vi "Pressure converstion.vi"(0 "Mod2/AI9":fxp<+/-,24,5>, 1 "Mod2/AI8":fxp<+/-,24,5>, 2 "Mod2/AI7":fxp<+/-,24,5>, 5 "Mod2/AI15":fxp<+/-,24,5>, 7 "Mod2/AI10":fxp<+/-,24,5>, 9 "Mod2/AI14":fxp<+/-,24,5>, 12 "Mod2/AI11":fxp<+/-,24,5>, 13 "Mod2/AI12":fxp<+/-,24,5>, 14 "Mod2/AI13":fxp<+/-,24,5>) -> (4 "P8 toP16":fxp<+/-,48,10>[](array[numeric]))   [LabVIEW 2018]
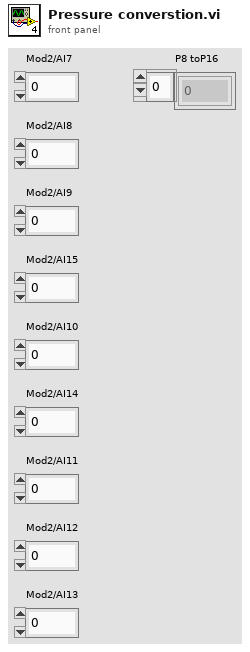
[diagram p1: front panel]
types:
  T1 = cluster{"Gain":fxp<+/-,24,5>, "offset":fxp<+/-,24,5>}
  T2 = cluster{"Gain":fxp<+/-,24,5>, "offset":fxp<+/-,24,5>, "offset 2":fxp<+/-,24,5>}
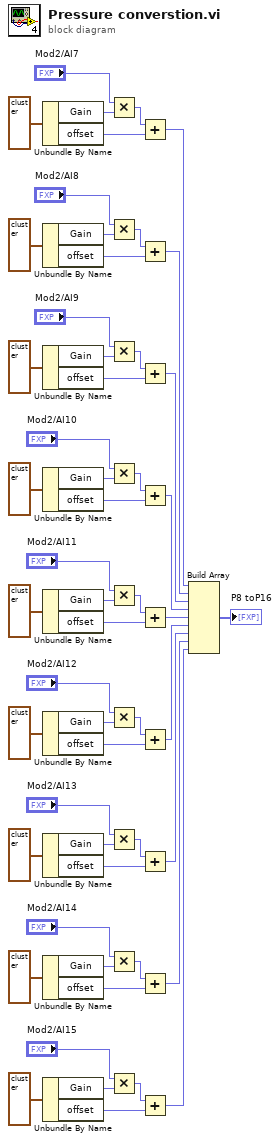
[diagram p0: block diagram]
diagram:
  n1 = Unbundle By Name(T1 {"Gain"=1.0, "offset"=0.0} ("Share_8_P")) -> ("Gain"=w25:fxp<+/-,24,5>, "offset"=w26:fxp<+/-,24,5>)
  n2 = Unbundle By Name(T1 {"Gain"=1.0, "offset"=0.0} ("Share_9_P")) -> ("Gain"=w27:fxp<+/-,24,5>, "offset"=w28:fxp<+/-,24,5>)
  n3 = Unbundle By Name(T1 {"Gain"=1.0, "offset"=0.0} ("Share_10_P")) -> ("Gain"=w29:fxp<+/-,24,5>, "offset"=w30:fxp<+/-,24,5>)
  n4 = Unbundle By Name(T1 {"Gain"=1.0, "offset"=0.0} ("Share_11_P")) -> ("Gain"=w31:fxp<+/-,24,5>, "offset"=w32:fxp<+/-,24,5>)
  n5 = Unbundle By Name(T1 {"Gain"=1.0, "offset"=0.0} ("Share_12_P")) -> ("Gain"=w33:fxp<+/-,24,5>, "offset"=w34:fxp<+/-,24,5>)
  n6 = Unbundle By Name(T1 {"Gain"=1.0, "offset"=0.0} ("Share_13_P")) -> ("Gain"=w35:fxp<+/-,24,5>, "offset"=w36:fxp<+/-,24,5>)
  n7 = Unbundle By Name(T2 {"Gain"=1.0, "offset"=0.0, "offset 2"=0.0} ("Share_14_P")) -> ("Gain"=w37:fxp<+/-,24,5>, "offset"=w38:fxp<+/-,24,5>)
  n8 = Unbundle By Name(T1 {"Gain"=1.0, "offset"=0.0} ("Share_15_P")) -> ("Gain"=w39:fxp<+/-,24,5>, "offset"=w40:fxp<+/-,24,5>)
  n9 = Unbundle By Name(T1 {"Gain"=1.0, "offset"=0.0} ("Share_15_P")) -> ("Gain"=w52:fxp<+/-,24,5>, "offset"=w53:fxp<+/-,24,5>)
  n10 = Multiply(x="Mod2/AI7", y=w25) -> (x*y=w15:fxp<+/-,48,10>)
  n11 = Multiply(x="Mod2/AI8", y=w27) -> (x*y=w14:fxp<+/-,48,10>)
  n12 = Multiply(x="Mod2/AI9", y=w29) -> (x*y=w13:fxp<+/-,48,10>)
  n13 = Multiply(x="Mod2/AI10", y=w31) -> (x*y=w12:fxp<+/-,48,10>)
  n14 = Multiply(x="Mod2/AI11", y=w33) -> (x*y=w11:fxp<+/-,48,10>)
  n15 = Multiply(x="Mod2/AI12", y=w35) -> (x*y=w10:fxp<+/-,48,10>)
  n16 = Multiply(x="Mod2/AI13", y=w37) -> (x*y=w9:fxp<+/-,48,10>)
  n17 = Multiply(x="Mod2/AI14", y=w39) -> (x*y=w23:fxp<+/-,48,10>)
  n18 = Multiply(x="Mod2/AI15", y=w52) -> (x*y=w49:fxp<+/-,48,10>)
  n19 = Add(x=w15, y=w26) -> (x+y=w41:fxp<+/-,48,10>)
  n20 = Add(x=w14, y=w28) -> (x+y=w42:fxp<+/-,48,10>)
  n21 = Add(x=w13, y=w30) -> (x+y=w43:fxp<+/-,48,10>)
  n22 = Add(x=w12, y=w32) -> (x+y=w44:fxp<+/-,48,10>)
  n23 = Add(x=w11, y=w34) -> (x+y=w45:fxp<+/-,48,10>)
  n24 = Add(x=w10, y=w36) -> (x+y=w46:fxp<+/-,48,10>)
  n25 = Add(x=w9, y=w38) -> (x+y=w47:fxp<+/-,48,10>)
  n26 = Add(x=w23, y=w40) -> (x+y=w48:fxp<+/-,48,10>)
  n27 = Add(x=w49, y=w53) -> (x+y=w54:fxp<+/-,48,10>)
  n28 = Build Array(w41, w42, w43, w44, w45, w46, w47, w48, w54) -> (→"P8 toP16":fxp<+/-,48,10>[])
